vi "DIAG_STM Write Message.vi"   [LabVIEW 2013, in "Diagnostics Addon Engine.lvlib"]
doc: "This VI writes a package of data to a remote computer. It prepends a meta data ID number to each packet. \n\nThe data must be passed in as a String. The calling VI is responsible for flattening the desired data to a string before passing it to this VI."
uses:
  Diagnostics Addon Engine.lvlib
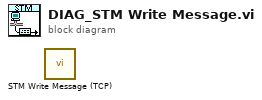
[diagram p0: block diagram]
diagram:
  n1 = call "STM Write Message (TCP).vi"() -> ()  [unwired: 10 in, 2 out]
